vi "DigitalOnOff.vi"(8 "error in (no error)":errorcluster, 10 "Parameters In":variant, 11 "Subpanel Queue In":refnum<queue>) -> (0 "error out":errorcluster, 2 "Parameters Out":variant)   [LabVIEW 2018]
doc: "Configuration control for the 'Hold' step."
panel:
  in  "Ligar?":bool caption="Configuration Control"
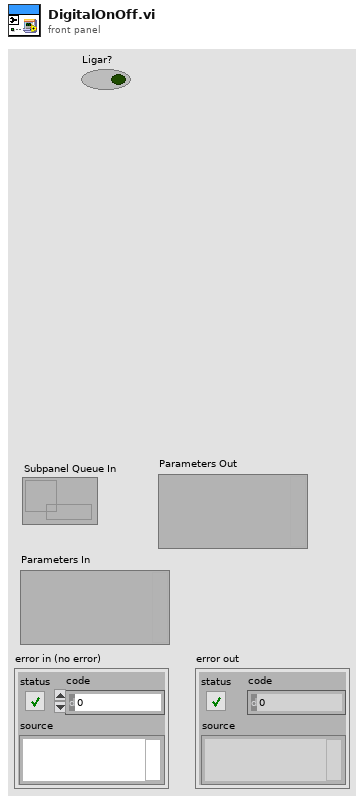
[diagram p1: front panel]
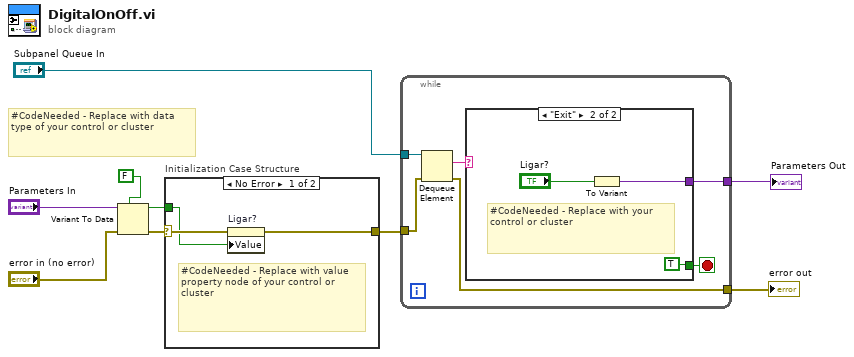
[diagram p0: block diagram]
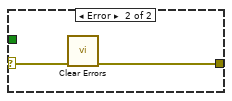
[diagram p2: hidden frame]
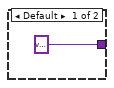
[diagram p3: hidden frame]
diagram:
  # "#CodeNeeded - Replace with data type of your control or cluster"
  n1 = Variant To Data(error in="error in (no error)", type=FALSE, Variant="Parameters In") -> (data=w7:bool, error out=w5:errorcluster)
  n2 = case "Initialization Case Structure" shown="No Error" w5 {
    selector: w5 -> [w12 w14]
    tunnel: w7 -> [w10 _]
    tunnel: [w11 w13] -> w6
    frame No Error {
      # "#CodeNeeded - Replace with value property node of your control or cluster"
      n3 = property on="Ligar?" class="Bool (strict)"(error in=w12, "Value"=w10) -> (error out=w11:errorcluster)  [unwired: 1 in, 1 out]
    }
    frame Error {
      n4 = call <vilib>:"Clear Errors.vi"("error in (no error)"=w14) -> ("error out"=w13:errorcluster)  [unwired: 5 in, 1 out]
    }
  }
  n5 = while {
    tunnel: "Subpanel Queue In" -> [w20]
    tunnel: w6 -> [w19]
    tunnel: [w17] -> w4
    tunnel: [w15] -> w2
    stop <- w16 stop-if-true
    n6 = Dequeue Element(queue=w20, error in (no error)=w19) -> (element=w18:string, error out=w15:errorcluster)  [unwired: 1 in, 2 out]
    n7 = case shown="\"Exit\"" w18 {
      tunnel: [variant ("Variant") w24] -> w17
      tunnel: [_ TRUE] -> w16
      frame Default {
      }
      frame "Exit" {
        # "#CodeNeeded - Replace with your control or cluster"
        n8 = To Variant(anything="Ligar?") -> (Variant=w24:variant)
      }
    }
  }
  "Parameters Out" <- w4
  "error out" <- w2
